vi "保险位置计算器.vi"(1 "保险位置":bool[][](array[boolean])) -> (0 "输出数组":i32[](array[numeric]))   [LabVIEW 2013]
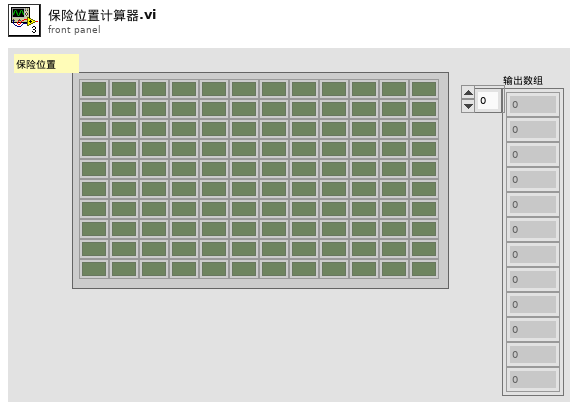
[diagram p1: front panel]
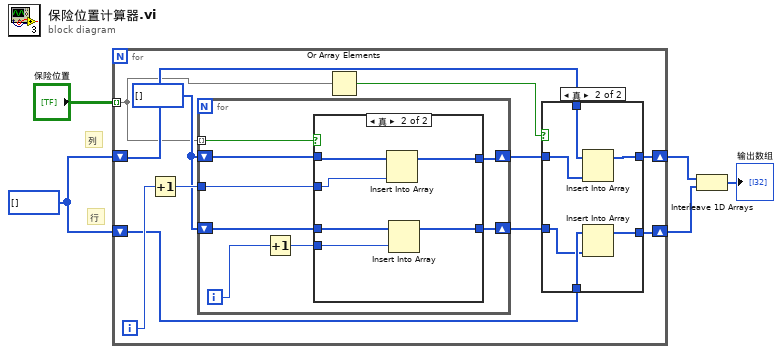
[diagram p0: block diagram]
diagram:
  w4 = i32[] []
  # "行"
  # "列"
  n1 = for {
    tunnel: "保险位置" -> [w8] mode=indexing
    shift-right: [w12] -> w3
    shift-left: w4 -> [w13]
    shift-right: [w10] -> w2
    shift-left: w4 -> [w9]
    i -> [w16]
    w14 = i32[] []
    n2 = Increment(x=w16) -> (x+1=w15:i32)
    n3 = for {
      tunnel: w8 -> [w32] mode=indexing
      tunnel: w15 -> [w30]
      shift-right: [w29] -> w6
      shift-left: w14 -> [w31]
      shift-right: [w26] -> w11
      shift-left: w14 -> [w27]
      i -> [w28]
      n4 = Increment(x=w28) -> (x+1=w25:i32)
      n5 = case shown="真" w32 {
        tunnel: w31 -> [w34 w40]
        tunnel: w30 -> [_ w39]
        tunnel: [w34 w38] -> w29
        tunnel: w25 -> [_ w36]
        tunnel: w27 -> [w33 w37]
        tunnel: [w33 w35] -> w26
        frame False {
        }
        frame True {
          n6 = Insert Into Array(array=w40, new element=w39) -> (w38:i32[])  [unwired: 1 in]
          n7 = Insert Into Array(array=w37, new element=w36) -> (w35:i32[])  [unwired: 1 in]
        }
      }
    }
    n8 = Or Array Elements(Boolean array=w8) -> (logical OR=w7:bool)
    n9 = case shown="真" w7 {
      tunnel: w6 -> [_ w24]
      tunnel: w13 -> [w18 w23]
      tunnel: [w18 w22] -> w12
      tunnel: w11 -> [_ w19]
      tunnel: [w17 w21] -> w10
      tunnel: w9 -> [w17 w20]
      frame False {
      }
      frame True {
        n10 = Insert Into Array(array=w23, new element=w24) -> (w22:i32[])  [unwired: 1 in]
        n11 = Insert Into Array(array=w20, new element=w19) -> (w21:i32[])  [unwired: 1 in]
      }
    }
  }
  n12 = Interleave 1D Arrays(w3, w2) -> (→"输出数组":i32[])
